vi "Check Disk Space.vi"(8 "error in (no error)":errorcluster, 10 "camera settings":T1={"Exposure Time (ms)"=100.0, "Binning"=enum."2x2", "Scan Mode"=-1, "Frames to Acquire"=1000.0, "Pixel Correction"=FALSE, "Frames to Skip"=1, "File Path"=path "", "Duty cycle"=1.0, "ALEX"=FALSE, "Shutter Enable"=[], "fluidics trigger frame"=0, "Bit Depth"=16, "Image Width (px)"=0, "Image Height (px)"=0, "Horizontal Offset (px)"=0, "Vertical Offset (px)"=0} {"Exposure Time (ms)" min=1.0 max=10000.0 step=1.0}, 11 "Camera in":refnum<class "Camera.lvclass">) -> (0 "error out":errorcluster, 2 "OK?":bool, 3 "Camera out":refnum<class "Camera.lvclass">)   [LabVIEW 2023, in "Camera.lvlib" / "Camera.lvclass"]
uses:
  Camera.lvclass
  Resources/Type Defs/Camera Settings.ctl
  Camera.lvclass/Camera.ctl
panel:
  out "space required (bytes)":i64 format="%.0e"
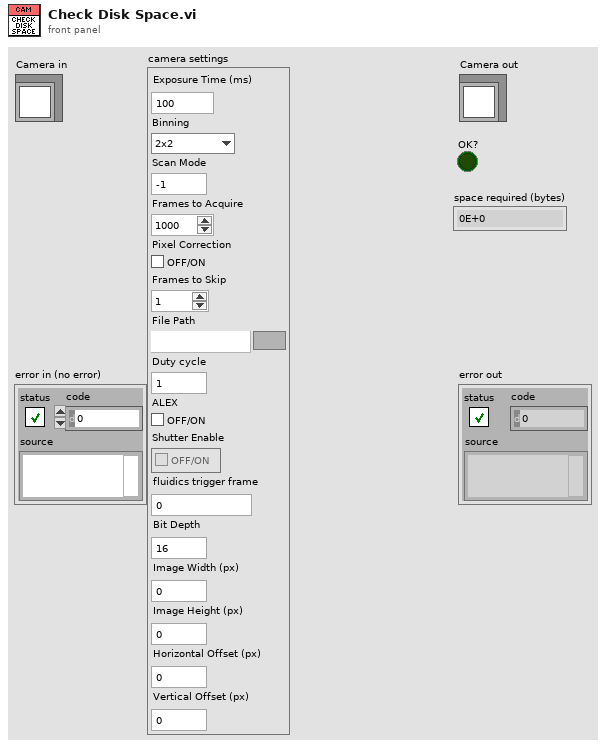
[diagram p1: front panel]
types:
  T1 = typedef "Camera Settings.ctl" = cluster{"Exposure Time (ms)":dbl, "Binning":enum16{"1x1", "2x2", "4x4"}, "Scan Mode":i32, "Frames to Acquire":dbl, "Pixel Correction":bool, "Frames to Skip":u32, "File Path":path, "Duty cycle":dbl, "ALEX":bool, "Shutter Enable":bool[], "fluidics trigger frame":u16, "Bit Depth":u16, "Image Width (px)":u16, "Image Height (px)":u16, "Horizontal Offset (px)":u16, "Vertical Offset (px)":u16}
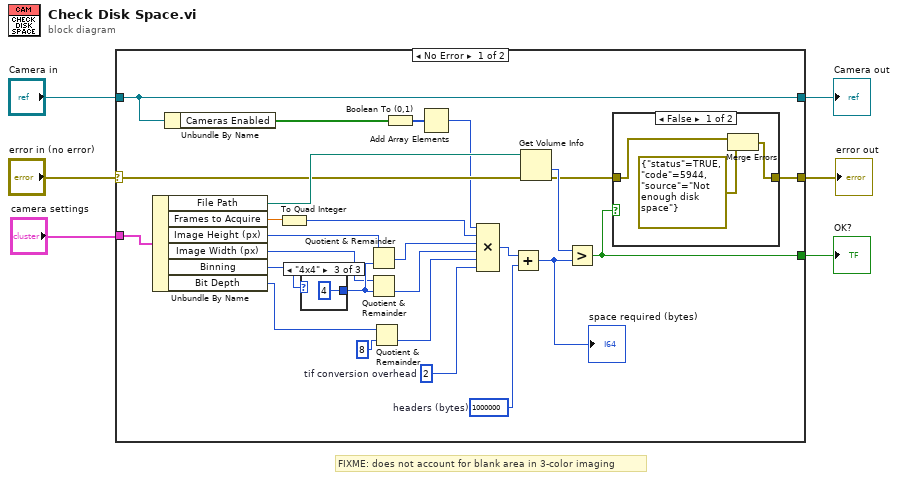
[diagram p0: block diagram]
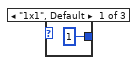
[diagram p2: hidden frame]
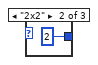
[diagram p3: hidden frame]
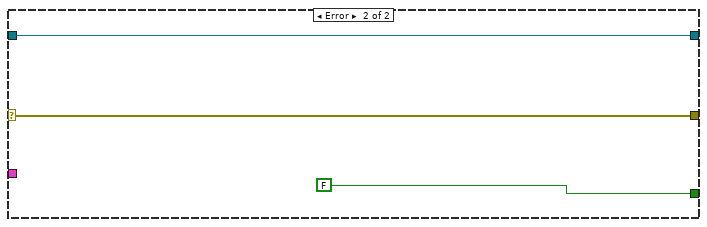
[diagram p5: hidden frame]
diagram:
  # "FIXME: does not account for blank area in 3-color imaging"
  n1 = case shown="No Error" "error in (no error)" {
    selector: "error in (no error)" -> [w26 w42]
    tunnel: "camera settings" -> [w28 _]
    tunnel: [w16 FALSE] -> w1
    tunnel: [w17 w42] -> w5
    tunnel: "Camera in" -> [w24 w40]
    tunnel: [w24 w40] -> w2
    frame No Error {
      w7 = i64 2  # tif conversion overhead
      w29 = i64 1000000  # headers (bytes)
      n2 = Unbundle By Name(w28) -> ("File Path"=w27:path, "Frames to Acquire"=w20:dbl, "Image Height (px)"=w15:u16, "Image Width (px)"=w12:u16, "Binning"=w10:enum16{"1x1", "2x2", "4x4"}, "Bit Depth"=w9:u16)
      n3 = Unbundle By Name(w24) -> ("Cameras Enabled"=w23:bool[])
      n4 = To Quad Integer(1:w20) -> (0:w19:i64)
      n5 = case shown="\"4x4\"" w10 {
        tunnel: [i64 1 ("y") i64 2 ("y") i64 4 ("y")] -> w13
        frame "1x1", Default {
        }
        frame "2x2" {
        }
        frame "4x4" {
        }
      }
      n6 = Quotient & Remainder(x=w15, y=w13) -> (floor(x/y)=w14:i64)  [unwired: 1 out]
      n7 = Quotient & Remainder(x=w12, y=w13) -> (floor(x/y)=w11:i64)  [unwired: 1 out]
      n8 = Quotient & Remainder(x=w9, y=i64 8) -> (floor(x/y)=w8:i64)  [unwired: 1 out]
      n9 = Boolean To (0,1)(Boolean=w23) -> (0, 1=w22:i16[])
      n10 = Add Array Elements(numeric array=w22) -> (sum=w21:i16)
      n11 = Compound Arithmetic op=MULTIPLY(w21, w19, w14, w11, w8, w7) -> (w31:i64)
      n12 = Add(x=w31, y=w29) -> (x+y=w32:i64)
      "space required (bytes)" <- w32
      n13 = Get Volume Info(8:w26, 11:w27) -> (0:w18:errorcluster, 1:w30:i64)  [unwired: 4 out]
      n14 = Greater?(x=w30, y=w32) -> (0:w16:bool)
      n15 = case shown="False" w16 {
        tunnel: w18 -> [w37 w39]
        tunnel: [w38 w39] -> w17
        frame False {
          n16 = Merge Errors(w37, errorcluster {"status"=TRUE, "code"=5944, "source"="Not enough disk space"} ("error in")) -> (w38:errorcluster)
        }
        frame True {
        }
      }
    }
    frame Error {
    }
  }
  "error out" <- w5
  "Camera out" <- w2
  "OK?" <- w1
